vi "Wave Memory Generator.vi"() -> (0 "FXP Init Data Out":fxp<+/-,12,12>[](array[numeric]), 3 "Init Data Out":i64[](array[numeric]))   [LabVIEW 2014]
uses:
  <vilib>/Utility/file.llb/Read From Spreadsheet File (I64).vi
  <vilib>/Analysis/NI_AALPro.lvlib
  <vilib>/Analysis/NI_AALBase.lvlib
panel:
  out "Frequency (Hz)":dbl
  out "Init Data Out Graph":i64[](graph)
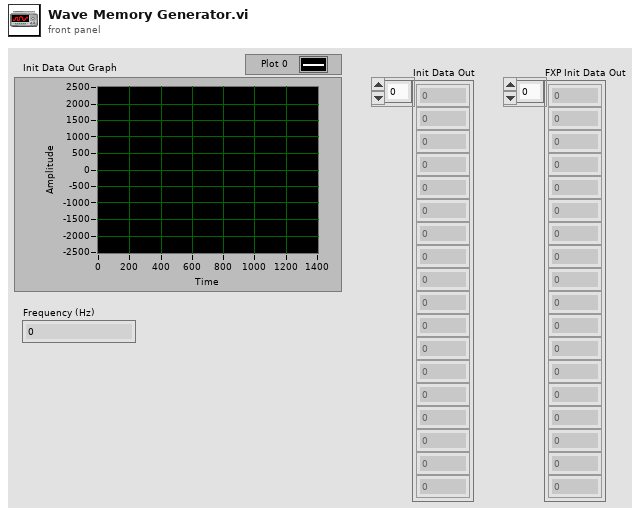
[diagram p1: front panel]
types:
  T1 = enum16{"sine", "cosine", "triangle", "square", "sawtooth", "increasing ramp", "decreasing ramp"}
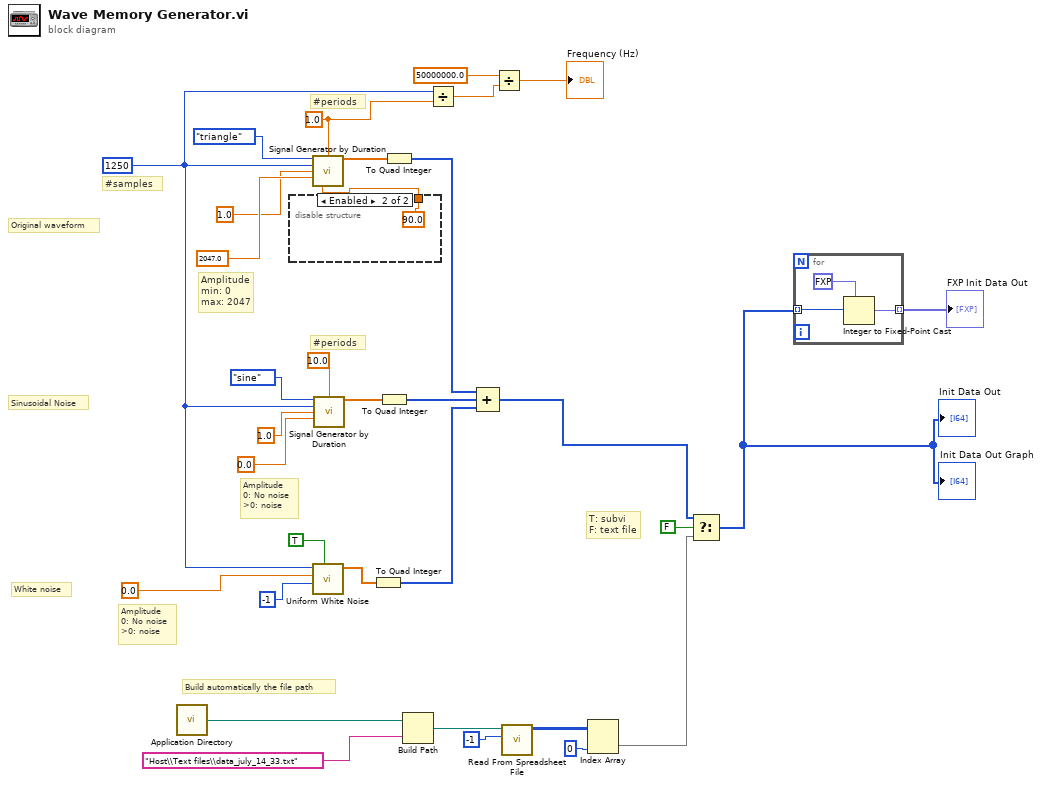
[diagram p0: block diagram]
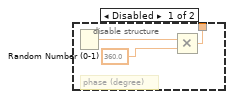
[diagram p2: hidden frame]
diagram:
  w14 = 1.0 ("duration")
  w15 = 1250 ("# of samples")
  # "T: subvi\nF: text file"
  # "Build automatically the file path"
  # "Amplitude\n0: No noise\n>0: noise"
  # "Original waveform"
  # "Sinusoidal Noise"
  # "White noise"
  # "#periods"
  # "Amplitude\n0: No noise\n>0: noise"
  # "#periods"
  # "Amplitude\nmin: 0\nmax: 2047"
  # "#samples"
  n1 = call <vilib>:"Application Directory.vi"() -> ("Application Directory"=w7:path)
  n2 = disable-structure shown="Enabled" {
    disable-tunnel: [w34 90.0 ("phase in")] -> w17
    frame Disabled {
      # "phase (degree)"
      n3 = Random Number (0-1)() -> (number: 0 to 1=w35:dbl)
      n4 = Multiply(x=w35, y=360.0) -> (x*y=w34:dbl)
    }
    frame Enabled {
    }
  }
  n5 = call <vilib>:"Signal Generator by Duration.vi"("signal type"=T1."triangle", "duration"=w14, "# of samples"=w15, "frequency"=1.0, "amplitude"=2047.0, "phase in"=w17) -> ("signal"=w19:dbl[])  [unwired: 6 in, 3 out]
  n6 = call <vilib>:"Uniform White Noise.vi"("initialize?"=TRUE, "seed"=-1, "amplitude"=0.0, "samples"=w15) -> ("uniform white noise"=w18:dbl[])  [unwired: 6 in, 1 out]
  n7 = call <vilib>:"Signal Generator by Duration.vi"("signal type"=T1."sine", "duration"=10.0, "# of samples"=w15, "frequency"=1.0, "amplitude"=0.0) -> ("signal"=w31:dbl[])  [unwired: 7 in, 3 out]
  n8 = To Quad Integer(1:w18) -> (0:w24:i64[])
  n9 = To Quad Integer(1:w31) -> (0:w26:i64[])
  n10 = To Quad Integer(1:w19) -> (0:w23:i64[])
  n11 = Build Path(base path=w7, name or relative path="Host\\Text files\\data_july_14_33.txt") -> (appended path=w5:path)
  n12 = Divide(x=w15, y=w14) -> (x/y=w13:dbl)
  n13 = Compound Arithmetic op=ADD(w23, w26, w24) -> (w2:i64[])
  n14 = Divide(x=50000000.0, y=w13) -> (x/y=→"Frequency (Hz)":dbl)
  n15 = call-poly <vilib>:"Read From Spreadsheet File.vi"("number of rows (all:-1)"=-1, "file path (dialog if empty)"=w5) -> ("all rows"=w9:i64[][])  [unwired: 5 in, 4 out]
  n16 = Index Array(array=w9, index (col)=0 ("disabled index (col)")) -> (element=w4:i64[])  [unwired: 1 in]
  n17 = Select(t=w2, s=FALSE, f=w4) -> (s? t:f=w1:i64[])
  "Init Data Out Graph" <- w1
  "Init Data Out" <- w1
  n18 = for {
    tunnel: w1 -> [w40] mode=indexing
    tunnel: [w38] -> w11 mode=indexing
    n19 = Integer to Fixed-Point Cast(fixed-point type=fxp<+/-,12,12> 0.0, integer=w40) -> (fixed-point=w38:fxp<+/-,12,12>)
  }
  "FXP Init Data Out" <- w11
